vi "convert_binData_to_floatArray.vi"(3 "Bin Float Number Format":T1, 5 "Bin Data":string) -> (0 "Array size":i32, 1 "Numbers out":dbl[](array[numeric]), 2 "Bin Data Aligned":bool)   [LabVIEW 2022 SP3, in "hmp4000_rsidr_core.lvlib"]
uses:
  hmp4000_rsidr_core.lvlib
  type_Binary_Float_Number_Format.ctl
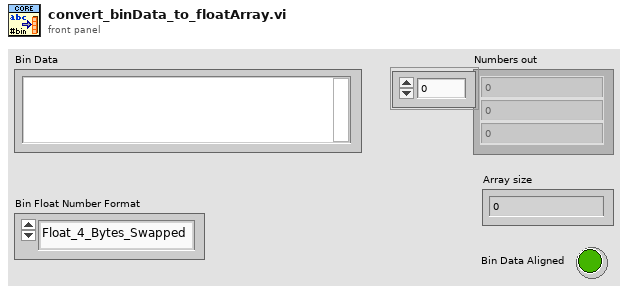
[diagram p1: front panel]
types:
  T1 = typedef "hmp4000_rsidr_core.lvlib/type_Binary_Float_Number_Format.ctl" = enum16{"Float_4_Bytes_Swapped", "Float_4_Bytes", "Double_8_Bytes_Swapped", "Double_8_Bytes"}
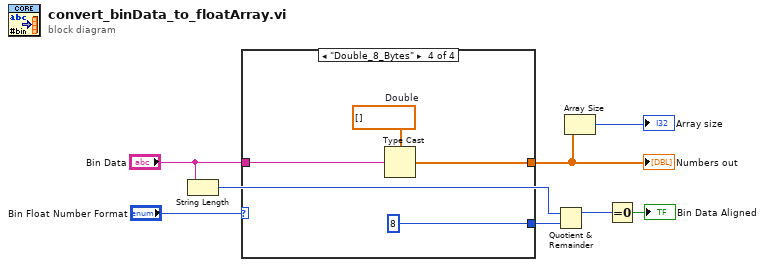
[diagram p0: block diagram]
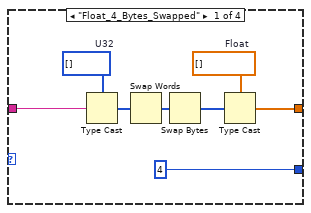
[diagram p2: hidden frame]
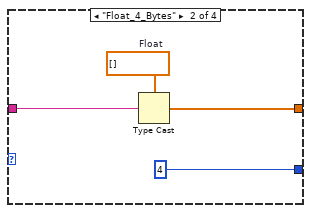
[diagram p3: hidden frame]
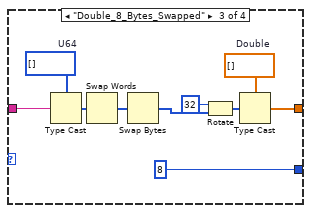
[diagram p4: hidden frame]
diagram:
  n1 = String Length(string="Bin Data") -> (length=w2:i32)
  n2 = case shown="\"Double_8_Bytes\"" "Bin Float Number Format" {
    tunnel: [w10 w18 w22 w32] -> w7
    tunnel: "Bin Data" -> [w11 w19 w23 w33]
    tunnel: [4 4 8 8] -> w1
    frame "Float_4_Bytes_Swapped" {
      w12 = u32[] []  # U32
      w13 = sgl[] []  # Float
      n3 = Type Cast(type=w12, x=w11) -> (*(type *) &x=w15:u32[])
      n4 = Swap Words(1:w15) -> (0:w14:u32[])
      n5 = Swap Bytes(anything=w14) -> (byte swapped=w16:u32[])
      n6 = Type Cast(type=w13, x=w16) -> (*(type *) &x=w10:sgl[])
    }
    frame "Float_4_Bytes" {
      w20 = sgl[] []  # Float
      n7 = Type Cast(type=w20, x=w19) -> (*(type *) &x=w18:sgl[])
    }
    frame "Double_8_Bytes_Swapped" {
      w29 = dbl[] []  # Double
      w30 = u64[] []  # U64
      n8 = Type Cast(type=w30, x=w23) -> (*(type *) &x=w26:u64[])
      n9 = Swap Words(1:w26) -> (0:w27:u64[])
      n10 = Swap Bytes(anything=w27) -> (byte swapped=w25:u64[])
      n11 = Rotate(1:w25, 2:i8 32 ("y")) -> (0:w24:u64[])
      n12 = Type Cast(type=w29, x=w24) -> (*(type *) &x=w22:dbl[])
    }
    frame "Double_8_Bytes" {
      w34 = dbl[] []  # Double
      n13 = Type Cast(type=w34, x=w33) -> (*(type *) &x=w32:dbl[])
    }
  }
  "Numbers out" <- w7
  n14 = Quotient & Remainder(x=w2, y=w1) -> (x-y*floor(x/y)=w5:i32)  [unwired: 1 out]
  n15 = Array Size(array=w7) -> (size(s)=→"Array size":i32)
  n16 = Equal To 0?(x=w5) -> (x = 0?=→"Bin Data Aligned":bool)
